vi "Write Roles.vi"(8 "error in (no error)":errorcluster, 10 "Roles":T1, 11 "KickPenaltyAllyPlay in":refnum<class "KickPenaltyAllyPlay.lvclass">) -> (0 "error out":errorcluster, 3 "KickPenaltyAllyPlay out":refnum<class "KickPenaltyAllyPlay.lvclass">)   [LabVIEW 2018, in "KickPenaltyAllyPlay.lvclass"]
uses:
  KickPenaltyAllyPlay.lvclass
  PenaltyAttackerRole_class/PenaltyAttackerRole.lvclass
  KickPenaltyAllyPlay.lvclass/KickPenaltyAllyPlay.ctl
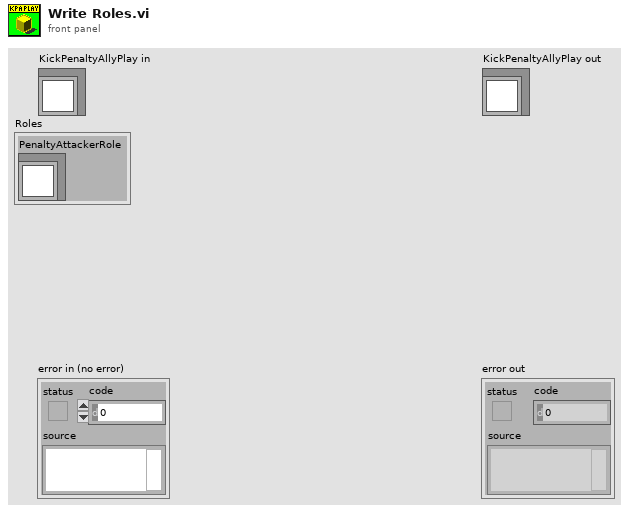
[diagram p1: front panel]
types:
  T1 = cluster{"PenaltyAttackerRole":refnum<class "PenaltyAttackerRole.lvclass">}
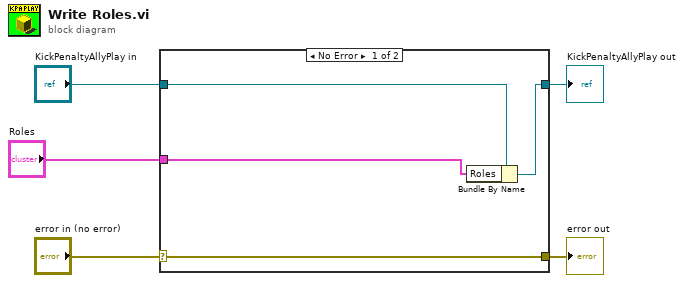
[diagram p0: block diagram]
diagram:
  n1 = case shown="No Error" "error in (no error)" {
    selector: "error in (no error)" -> [w9 w10]
    tunnel: [w9 w10] -> w4
    tunnel: [w7 w11] -> w2
    tunnel: "KickPenaltyAllyPlay in" -> [w8 w11]
    tunnel: "Roles" -> [w6 _]
    frame No Error {
      n2 = Bundle By Name(cluster=w8, "Roles"=w6) -> (w7:refnum<class "KickPenaltyAllyPlay.lvclass">)
    }
    frame Error {
    }
  }
  "error out" <- w4
  "KickPenaltyAllyPlay out" <- w2
